vi "Belkin IP Acq and Center Finder.vi"(5 "Reset":bool, 7 "Color Plane":i32(ring)=1 items=["Red", "Green", "Blue", "Hue", "Saturation", "Luminance", "Value", "Intensity"], 8 "error in (no error)":errorcluster, 9 "Threshold Limits":cluster{"Lower value":sgl, "Upper value":sgl}={"Lower value"=0.0, "Upper value"=255.0}, 10 "Image Dst":T2, 11 "ImageIn":T2) -> (0 "X":u16, 1 "ImgOut":T2, 2 "Y":u16, 4 "timing":T1, 6 "threshold":sgl)   [LabVIEW 2015]
uses:
  <vilib>/vision/Image Controls.llb/IMAQ Image.ctl
  Stream/LP Globals.vi
  <vilib>/vision/NI_Vision_Development_Module.lvlib
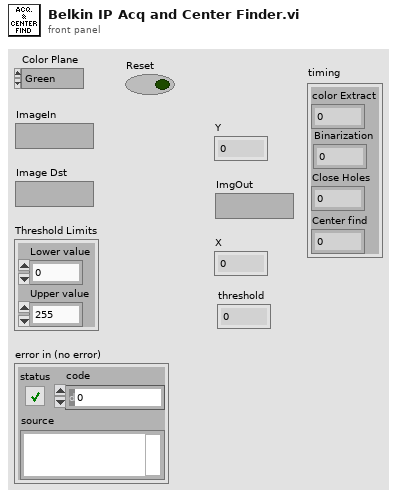
[diagram p1: front panel]
types:
  T1 = cluster{"color Extract":u32, "Binarization":u32, "Close Holes":u32, "Center find":u32}
  T2 = typedef "IMAQ Image.ctl" = refnum<image>
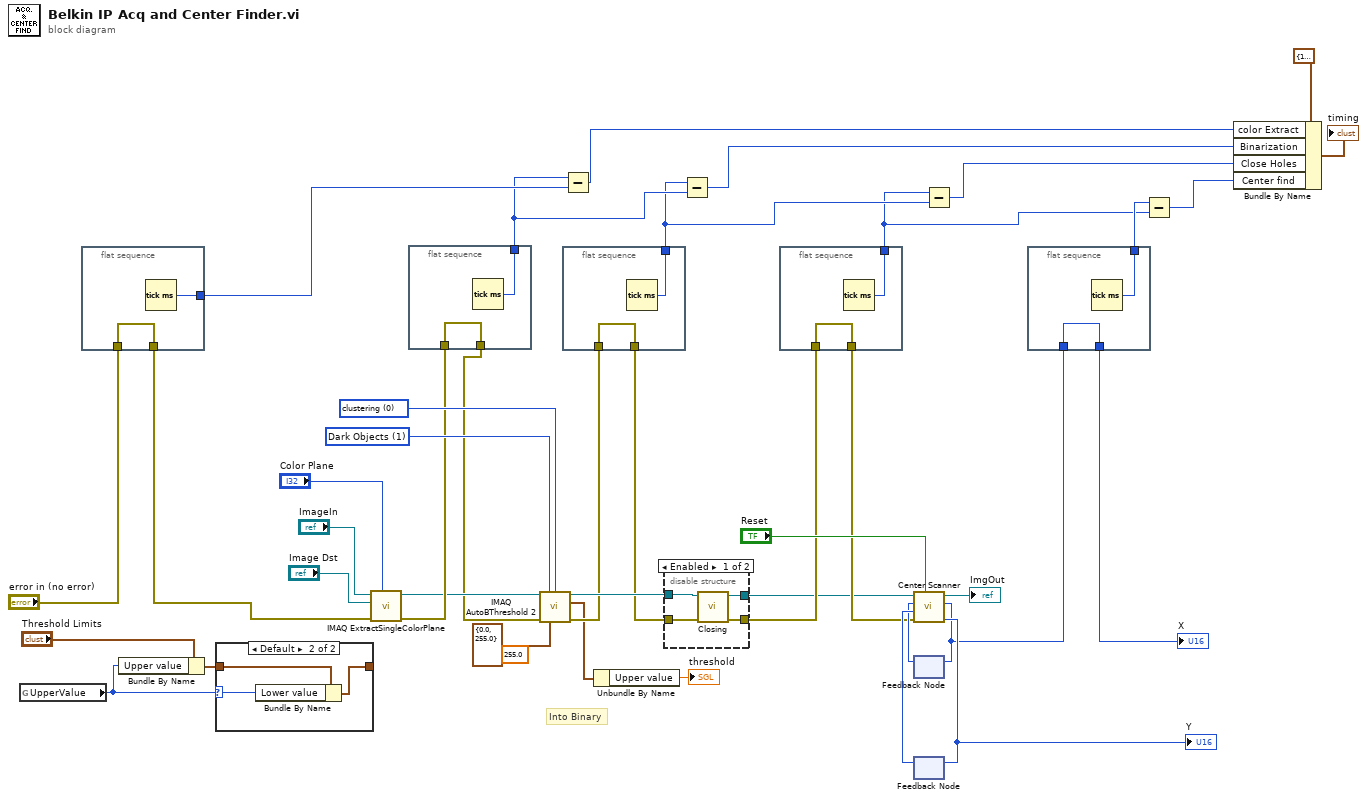
[diagram p0: block diagram]
diagram:
  (unwired) sgl 255.0 ("Replace Value (1)")
  w39 = u32 1 items=["Bright Objects", "Dark Objects"] ("Look For (Bright Objects)")
  w38 = 0 items=["clustering", "entropy", "metric", "moments", "inter-class variance"] ("Method")
  # "Into Binary"
  n1 = global read "LP Globals.vi" "UpperValue"() -> (w36:u8)
  n2 = flat-sequence {
    tunnel: "error in (no error)" -> [w42]
    tunnel: [w42] -> w26
    tunnel: [w41] -> w18
    frame #0 {
      n3 = Tick Count (ms)() -> (millisecond timer value=w41:u32)
    }
  }
  n4 = Bundle By Name(cluster="Threshold Limits", "Upper value"=w36) -> (w35:cluster{"Lower value":sgl, "Upper value":sgl})
  n5 = case shown="Default" w36 {
    selector: w36 -> [_ w44]
    tunnel: w35 -> [w43 w46]
    tunnel: [w43 w45] -> _
    frame 255 {
    }
    frame Default {
      n6 = Bundle By Name(cluster=w46, "Lower value"=w44) -> (w45:cluster{"Lower value":sgl, "Upper value":sgl})
    }
  }
  n7 = call "IMAQ ExtractSingleColorPlane"("Color Plane"="Color Plane", "error in (no error)"=w26, "Image Dst"="Image Dst", "Image Src"="ImageIn") -> ("error out"=w25:errorcluster, "Image Dst Out"=w2:T2)  [unwired: 6 out]
  n8 = flat-sequence {
    tunnel: w25 -> [w48]
    tunnel: [w48] -> w1
    tunnel: [w47] -> w17
    frame #0 {
      n9 = Tick Count (ms)() -> (millisecond timer value=w47:u32)
    }
  }
  n10 = call "IMAQ AutoBThreshold 2"("Image Src"=w2, "Look For (Bright Objects)"=w39, "Method (clustering)"=w38, "error in (no error)"=w1, "Threshold Limits"=cluster{"Lower value":sgl, "Upper value":sgl} {"Lower value"=0.0, "Upper value"=255.0}) -> ("Image Dst Out"=w40:T2, "Threshold Range Out"=w7:cluster{"Lower value":sgl, "Upper value":sgl}, "error out"=w24:errorcluster)  [unwired: 3 in, 5 out]
  n11 = Subtract(x=w17, y=w18) -> (x-y=w11:u32)
  n12 = flat-sequence {
    tunnel: w24 -> [w50]
    tunnel: [w50] -> w23
    tunnel: [w49] -> w16
    frame #0 {
      n13 = Tick Count (ms)() -> (millisecond timer value=w49:u32)
    }
  }
  n14 = Unbundle By Name(w7) -> ("Upper value"=→"threshold":sgl)
  n15 = disable-structure shown="Enabled" {
    disable-tunnel: w40 -> [w54 w56]
    disable-tunnel: [w53 w56] -> w3
    disable-tunnel: w23 -> [w52 w55]
    disable-tunnel: [w51 w55] -> w22
    frame Enabled {
      n16 = call "Closing.vi"("error in (no error)"=w52, "Refnum in"=w54) -> ("error out"=w51:errorcluster, "Refnum out"=w53:T2)  [unwired: 8 in]
    }
    frame Disabled {
    }
  }
  n17 = Subtract(x=w16, y=w17) -> (x-y=w10:u32)
  n18 = flat-sequence {
    tunnel: w22 -> [w58]
    tunnel: [w58] -> w21
    tunnel: [w57] -> w14
    frame #0 {
      n19 = Tick Count (ms)() -> (millisecond timer value=w57:u32)
    }
  }
  n20 = feedback #1() -> (w28:u16)  [unwired: 1 in]
  n21 = feedback #2() -> (w29:u16)  [unwired: 1 in]
  n22 = call "Center Scanner.vi"("Reset"="Reset", "error in (no error)"=w21, "PrevY"=w29, "PrevX"=w28, "Refnum in"=w3) -> ("Y"=w30:u16, "X"=w20:u16, "Refnum out"=→"ImgOut":T2)  [unwired: 4 in]
  "Y" <- w30
  n23 = feedback-in #1(w20) -> ()
  n24 = feedback-in #2(w30) -> ()
  n25 = Subtract(x=w14, y=w16) -> (x-y=w9:u32)
  n26 = flat-sequence {
    tunnel: w20 -> [w60]
    tunnel: [w60] -> w19
    tunnel: [w59] -> w15
    frame #0 {
      n27 = Tick Count (ms)() -> (millisecond timer value=w59:u32)
    }
  }
  n28 = Subtract(x=w15, y=w14) -> (x-y=w8:u32)
  n29 = Bundle By Name(cluster=T1 {"color Extract"=19, "Binarization"=2, "Close Holes"=427, "Center find"=253} ("timing"), "color Extract"=w11, "Binarization"=w10, "Close Holes"=w9, "Center find"=w8) -> (→"timing":T1)
  "X" <- w19
